vi "Go_to_Deposit.vi"(8 "error in (no error)":errorcluster, 11 "User_Console in":refnum<class "User_Console.lvclass">) -> (0 "error out":errorcluster, 3 "State out":refnum<class "State Actor.lvclass">)   [LabVIEW 2025, in "User_Console.lvlib" / "User_Console.lvclass"]
uses:
  User_Console.lvclass
  User_Console.lvclass/User_Console.ctl
  C:/Program Files (x86)/National Instruments/LabVIEW 2025/vi.lib/ni/Actors/State Actor/State Actor/State Actor.lvclass
  C:/Program Files (x86)/National Instruments/LabVIEW 2025/vi.lib/ActorFramework/Actor/Actor.lvclass
  C:/Users/halstead_rideriver/Documents/Labview_Practice/ATM_Machine_Actor Framework/ATM_ACTORFW/User_Console/User_Console/User_Console.lvclass
  Deposit/Deposit.lvclass
  C:/Users/halstead_rideriver/Documents/Labview_Practice/ATM_Machine_Actor Framework/ATM_ACTORFW/User_Console/Deposit/Deposit.lvclass
  <vilib>/ni/Actors/State Actor/State Actor/State Actor.lvclass
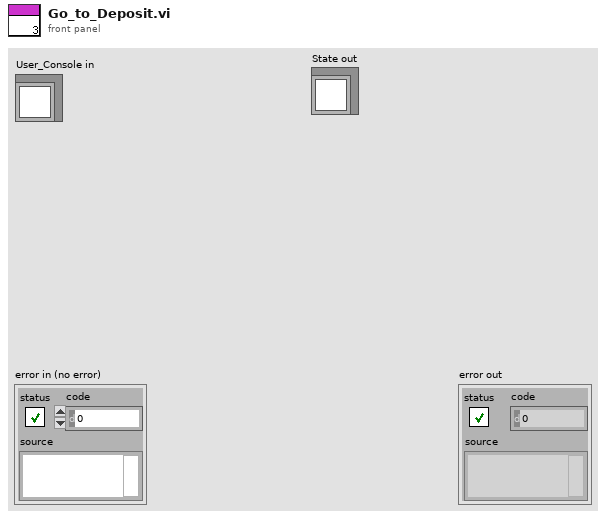
[diagram p1: front panel]
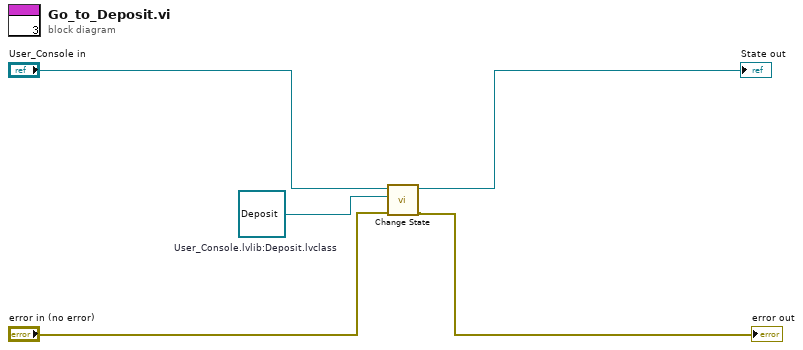
[diagram p0: block diagram]
diagram:
  w1 = refnum<class "Deposit.lvclass"> refnum  # User_Console.lvlib:Deposit.lvclass
  n1 = call <vilib>:"Change State.vi"("error in (no error)"="error in (no error)", "New State in"=w1, "State in"="User_Console in") -> ("error out"=→"error out":errorcluster, "State out"=→"State out":refnum<class "State Actor.lvclass">)  [unwired: 7 in]
